vi "Example.vi"(3 "stop":bool) -> (1 "error out":errorcluster)   [LabVIEW 2022 SP3, in "Logger.lvlib"]
uses:
  Logger.lvlib
  Logger/_Level.ctl
  FileHandler/FileHandler.lvclass
  C:/Users/jakub/repos/gh/sw4sys/lv-logger/Logger/Source/Handler/Handler.lvclass
  Logger/Logger.lvclass
  DateTime/Source/DateTime.lvlib
  Handler/Handler.lvclass
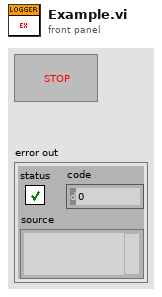
[diagram p1: front panel]
types:
  T1 = typedef "Logger.lvlib/Logger.lvclass/_Level.ctl" = enum16{"NOTSET", "DEBUG", "INFO", "WARNING", "ERROR", "CRITICAL"}
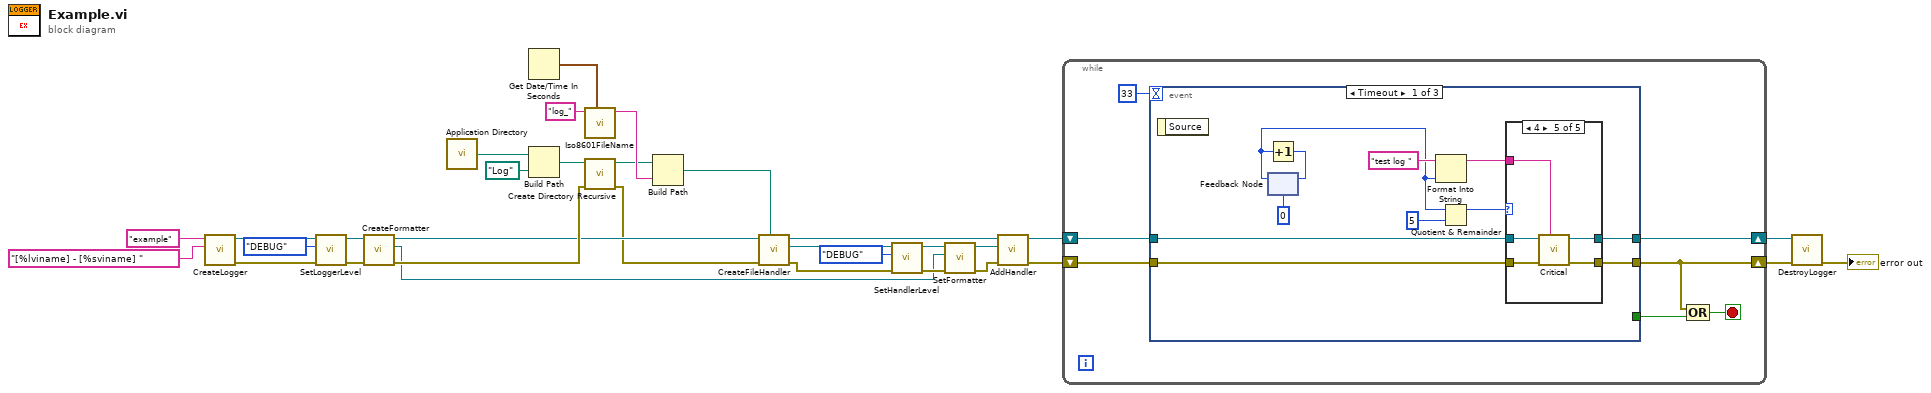
[diagram p0: block diagram]
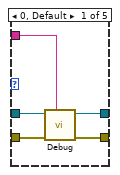
[diagram p2: hidden frame]
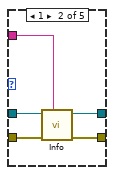
[diagram p3: hidden frame]
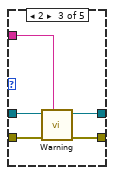
[diagram p4: hidden frame]
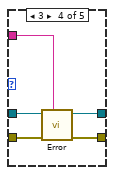
[diagram p5: hidden frame]
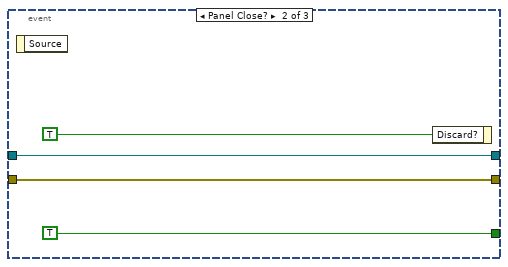
[diagram p6: hidden frame]
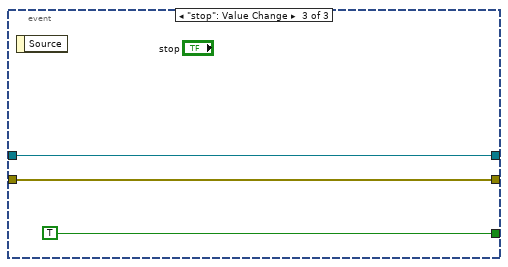
[diagram p7: hidden frame]
diagram:
  n1 = call "CreateLogger.vi"("MessagePrefixFormat"="[%lviname] - [%sviname] ", "Name"="example") -> ("error out"=w32:errorcluster, "Logger"=w24:refnum<class "Logger.lvclass">)  [unwired: 8 in]
  n2 = call-dynamic "SetLoggerLevel.vi"("error in (no error)"=w32, "Level"=_Level."DEBUG", "Logger in"=w24) -> ("error out"=w25:errorcluster, "Logger out"=w20:refnum<class "Logger.lvclass">)  [unwired: 7 in]
  n3 = call-dynamic "CreateFormatter.vi"("error in (no error)"=w25, "Logger in"=w20) -> ("error out"=w17:errorcluster, "Formatter"=w4:refnum<class "Formatter.lvclass">, "Logger out"=w12:refnum<class "Logger.lvclass">)  [unwired: 7 in]
  n4 = call <vilib>:"Application Directory.vi"() -> ("Application Directory"=w29:path)
  n5 = Get Date/Time In Seconds() -> (seconds since 1Jan1904=w6:timestamp)
  n6 = Build Path(base path=w29, name or relative path=path "Log") -> (appended path=w15:path)
  n7 = call "Iso8601FileName.vi"("TimeStamp"=w6, "Prefix ('')"="log_") -> ("FileName"=w14:string)  [unwired: 9 in]
  n8 = call <vilib>:"Create Directory Recursive.vi"("error in (no error)"=w17, "directory"=w15) -> ("error out"=w11:errorcluster, "directory copy"=w5:path)  [unwired: 3 in, 1 out]
  n9 = Build Path(base path=w5, name or relative path=w14) -> (appended path=w13:path)
  n10 = call-dynamic "CreateFileHandler.vi"("FIlePath"=w13, "error in (no error)"=w11, "Logger in"=w12) -> ("error out"=w30:errorcluster, "FileHandler"=w10:refnum<class "FileHandler.lvclass">, "Logger out"=w8:refnum<class "Logger.lvclass">)  [unwired: 6 in]
  n11 = call "SetHandlerLevel.vi"("error in (no error)"=w30, "Level"=_Level."DEBUG", "Handler in"=w10) -> ("error out"=w26:errorcluster, "Handler out"=w9:refnum<class "Handler.lvclass">)  [unwired: 7 in]
  n12 = call "SetFormatter.vi"("error in (no error)"=w26, "Formatter in"=w4, "Handler in"=w9) -> ("error out"=w19:errorcluster, "Handler out"=w18:refnum<class "Handler.lvclass">)  [unwired: 6 in, 1 out]
  n13 = call-dynamic "AddHandler.vi"("error in (no error)"=w19, "Handler in"=w18, "Logger in"=w8) -> ("error out"=w22:errorcluster, "Logger out"=w21:refnum<class "Logger.lvclass">)  [unwired: 6 in, 1 out]
  n14 = while {
    shift-right: [w37] -> w27
    shift-left: w21 -> [w39]
    shift-right: [w33] -> w28
    shift-left: w22 -> [w38]
    stop <- w35 stop-if-true
    n15 = event shown="[0] Timeout" {
      selector: _ -> [_ _ _]
      dyn-events: _ -> [_ _ _]
      timeout: 33 ("millisecond multiple") -> [_ _ _]
      tunnel: w39 -> [w50 w78 w82]
      tunnel: w38 -> [w49 w77 w81]
      tunnel: [w48 w78 w82] -> w37
      tunnel: [_ TRUE ("stop") TRUE ("stop")] -> w36
      tunnel: [w46 w77 w81] -> w33
      event Timeout {
        n16 = event-data() -> ()  [unwired: 1 in, 1 out]
        n17 = feedback #1(u32 0) -> (w40:u32)
        n18 = Increment(x=w40) -> (x+1=w41:u32)
        n19 = feedback-in #1(w41) -> ()
        n20 = Format Into String(initial string="test log ", w40) -> (resulting string=w43:string)  [unwired: 2 in, 1 out]
        n21 = Quotient & Remainder(x=w40, y=u32 5) -> (x-y*floor(x/y)=w44:u32)  [unwired: 1 out]
        n22 = case shown="4" w44 {
          tunnel: w50 -> [w53 w60 w63 w68 w73]
          tunnel: w49 -> [w55 w59 w65 w70 w75]
          tunnel: [w52 w58 w62 w67 w72] -> w48
          tunnel: [w54 w57 w64 w69 w74] -> w46
          tunnel: w43 -> [w51 w56 w61 w66 w71]
          frame 0, Default {
            n23 = call-dynamic "Debug.vi"("Message"=w51, "error in (no error)"=w55, "Logger in"=w53) -> ("error out"=w54:errorcluster, "Logger out"=w52:refnum<class "Logger.lvclass">)  [unwired: 7 in]
          }
          frame 1 {
            n24 = call-dynamic "Info.vi"("Message"=w56, "error in (no error)"=w59, "Logger in"=w60) -> ("error out"=w57:errorcluster, "Logger out"=w58:refnum<class "Logger.lvclass">)  [unwired: 7 in]
          }
          frame 2 {
            n25 = call-dynamic "Warning.vi"("Message"=w61, "error in (no error)"=w65, "Logger in"=w63) -> ("error out"=w64:errorcluster, "Logger out"=w62:refnum<class "Logger.lvclass">)  [unwired: 7 in]
          }
          frame 3 {
            n26 = call-dynamic "Error.vi"("Message"=w66, "error in (no error)"=w70, "Logger in"=w68) -> ("error out"=w69:errorcluster, "Logger out"=w67:refnum<class "Logger.lvclass">)  [unwired: 7 in]
          }
          frame 4 {
            n27 = call-dynamic "Critical.vi"("Message"=w71, "error in (no error)"=w75, "Logger in"=w73) -> ("error out"=w74:errorcluster, "Logger out"=w72:refnum<class "Logger.lvclass">)  [unwired: 7 in]
          }
        }
      }
      event Panel Close? {
        n28 = event-data() -> ()  [unwired: 1 in, 1 out]
        n29 = event-data("Discard?"=TRUE) -> ()  [unwired: 1 in, 1 out]
      }
      event "stop": Value Change {
        n30 = event-data() -> ()  [unwired: 1 in, 1 out]
      }
    }
    n31 = Compound Arithmetic op=OR(w33, w36) -> (w35:bool)
  }
  n32 = call-dynamic "DestroyLogger.vi"("error in (no error)"=w28, "Logger in"=w27) -> ("error out"=→"error out":errorcluster)  [unwired: 9 in]
